vi "TDMS Numeric 2D Array to file.vi"(0 "Base path":path, 1 "Group Name":string="A", 2 "FileName":string, 3 "Interval":T1=enum."Daily", 5 "Channel Names":string[](array[string]), 9 "2D array":dbl[][](array[numeric]), 11 "error in (no error)":errorcluster, 12 "Channel Units":string[](array[string]), 13 "property Metadata":variant[](array[variant])) -> (4 "file out":refnum<k34>, 15 "error out":errorcluster)   [LabVIEW 2019]
doc: "This SubVI manages the TDMS write process for data formatted into string arrays. On first run or after a specified interval, it will create a new TDMS file with a unique file name utilizing the data and time when the file is created. During the first run, it will populate the metadata and unit fields of the TDMS header. After a specified interval of data streaming to the file, it will be closed and the file extension will be changed from .tdms to .done. This is feature is to assure file transfer functions don't grab files that are being actively written to (LabVIEW's TDMS Open vi does not allow custom/alternate/temp file extensions). File write buffers are automatically flushed every 60 seconds to assure minimal data loss in the event of a power failure or program interruption. \n\n\nThis vi differs from version 1 by adding inputs for writing to the units column in the metadata page. Will replace version 1 once other code is updated.\n\n2020 NREL"
uses:
  Enum_FileNewInterval.ctl
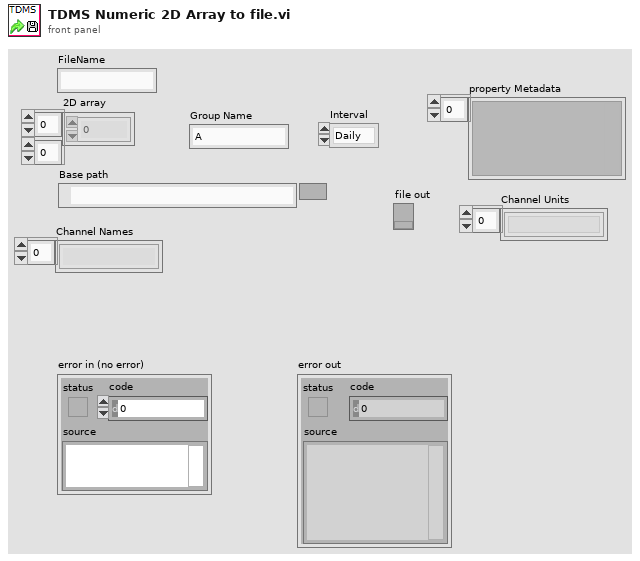
[diagram p1: front panel]
types:
  T1 = typedef "Enum_FileNewInterval.ctl" = enum16{"10 Min", "Hourly", "Daily", "Weekly", "Monthly"}
  T2 = enum16{"open", "open or create", "create or replace", "create", "open (read-only)"}
  T3 = typedef "LVDateTimeRec.ctl" = cluster{"fractional second":dbl, "second":i32, "minute":i32, "hour":i32, "day of month":i32, "month":i32, "year":i32, "day of week":i32, "day of year":i32, "DST":i32}
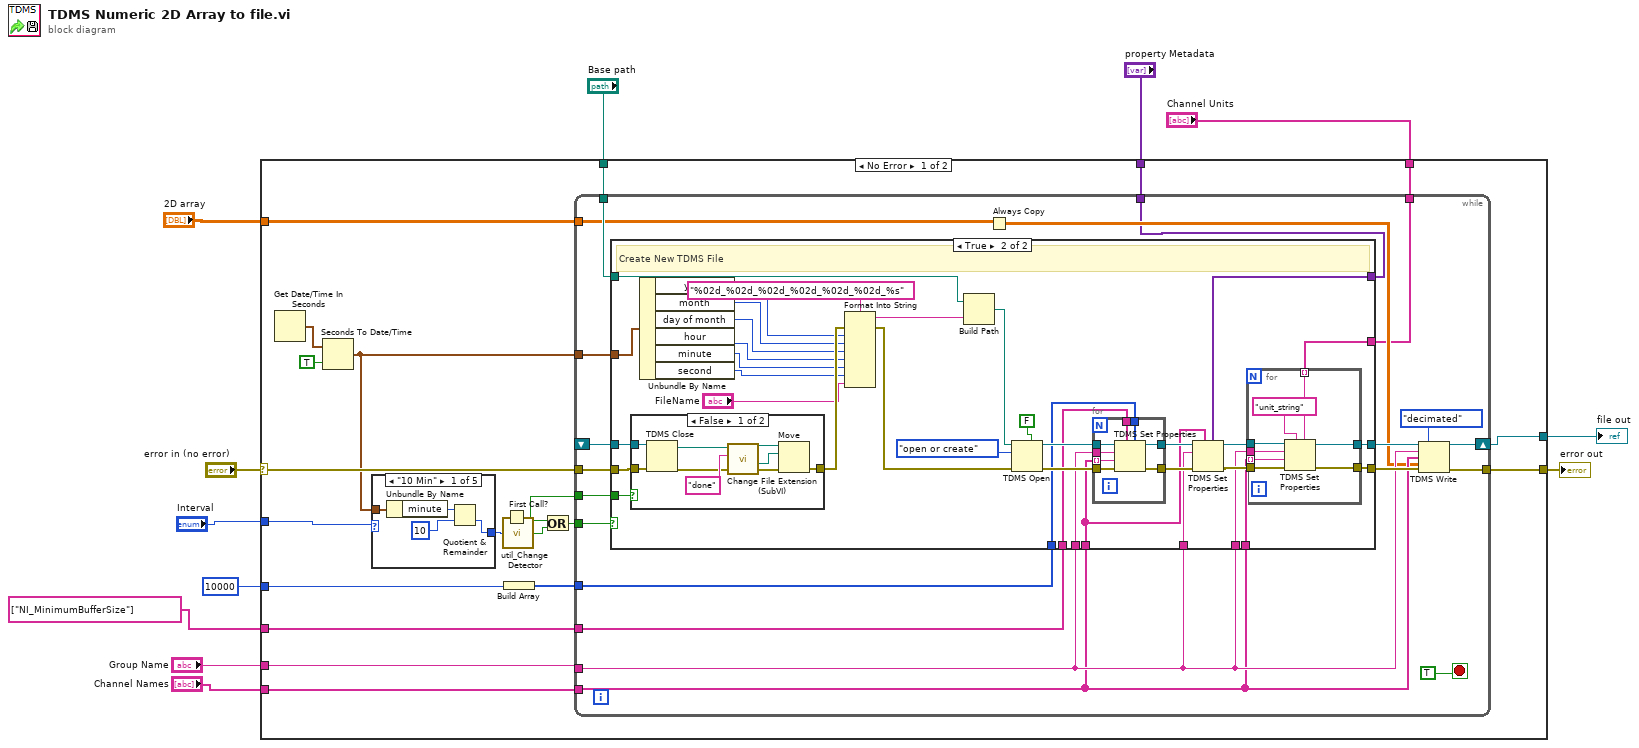
[diagram p0: block diagram]
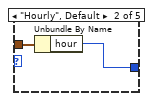
[diagram p2: hidden frame]
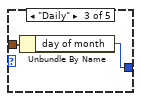
[diagram p3: hidden frame]
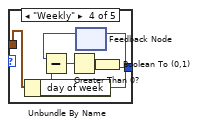
[diagram p4: hidden frame]
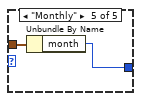
[diagram p5: hidden frame]
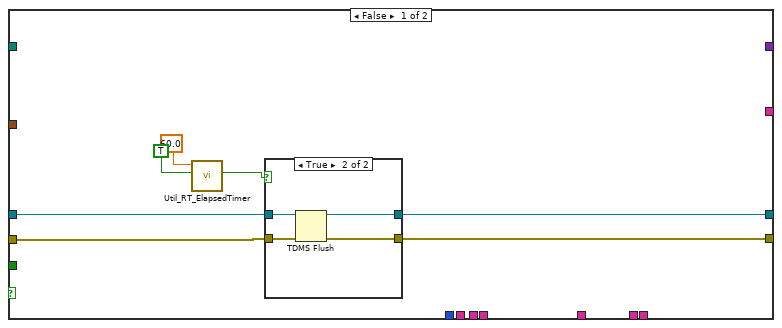
[diagram p6: hidden frame]
diagram:
  n1 = case shown="No Error" "error in (no error)" {
    selector: "error in (no error)" -> [w29 w143]
    tunnel: [w30 w143] -> w12
    tunnel: 10000 -> [w22 _]
    tunnel: "Interval" -> [w21 _]
    tunnel: string[] ["NI_MinimumBufferSize"] ("Channel Names") -> [w20 _]
    tunnel: "Channel Names" -> [w19 _]
    tunnel: "Group Name" -> [w18 _]
    tunnel: "Channel Units" -> [w17 _]
    tunnel: "property Metadata" -> [w16 _]
    tunnel: "Base path" -> [w15 _]
    tunnel: [w14 _] -> w2
    tunnel: "2D array" -> [w13 _]
    frame No Error {
      n2 = Get Date/Time In Seconds() -> (seconds since 1Jan1904=w26:timestamp)
      n3 = Seconds To Date/Time(time stamp (now)=w26, to UTC (F)=TRUE) -> (date time rec=w25:T3)
      n4 = case shown="\"10 Min\"" w21 {
        tunnel: w25 -> [w36 w38 w40 w46 w48]
        tunnel: [w33 w37 w39 w41 w47] -> w23
        frame "10 Min" {
          n5 = Unbundle By Name(w36) -> ("minute"=w35:i32)
          n6 = Quotient & Remainder(x=w35, y=10) -> (floor(x/y)=w33:i32)  [unwired: 1 out]
        }
        frame "Hourly", Default {
          n7 = Unbundle By Name(w38) -> ("hour"=w37:i32)
        }
        frame "Daily" {
          n8 = Unbundle By Name(w40) -> ("day of month"=w39:i32)
        }
        frame "Weekly" {
          n9 = Unbundle By Name(w46) -> ("day of week"=w44:i32)
          n10 = feedback-in #1(w44) -> ()
          n11 = feedback #1() -> (w45:i32)  [unwired: 1 in]
          n12 = Subtract(x=w45, y=w44) -> (x-y=w43:i32)
          n13 = Greater Than 0?(x=w43) -> (x > 0?=w42:bool)
          n14 = Boolean To (0,1)(Boolean=w42) -> (0, 1=w41:i16)
        }
        frame "Monthly" {
          n15 = Unbundle By Name(w48) -> ("month"=w47:i32)
        }
      }
      n16 = First Call?() -> (First Call?: T/F=w31:bool)
      n17 = call "util_Change Detector.vi"("value"=w23) -> ("changed?"=w24:bool)
      n18 = Build Array(w22) -> (w28:i32[])
      n19 = Or(x=w31, y=w24) -> (x .or. y?=w32:bool)
      n20 = while {
        tunnel: w32 -> [w68]
        shift-right: [w66] -> w14
        shift-left: _ -> [w67]
        tunnel: w31 -> [w65]
        tunnel: [w63] -> w30
        tunnel: w29 -> [w62]
        tunnel: w25 -> [w60]
        tunnel: w28 -> [w59]
        tunnel: w18 -> [w56]
        tunnel: w19 -> [w55]
        tunnel: w20 -> [w53]
        tunnel: w17 -> [w52]
        tunnel: w16 -> [w51]
        tunnel: w15 -> [w50]
        tunnel: w13 -> [w49]
        stop <- TRUE stop-if-true
        n21 = case shown="True" w68 {
          tunnel: w67 -> [w75 w112]
          tunnel: w65 -> [_ w113]
          tunnel: [w72 w90] -> w58
          tunnel: w62 -> [w73 w111]
          tunnel: w60 -> [_ w109]
          tunnel: [w74 w91] -> w57
          tunnel: w59 -> [_ w106]
          tunnel: w53 -> [_ w105]
          tunnel: w56 -> [_ w93]
          tunnel: w55 -> [_ w96]
          tunnel: w56 -> [_ w95]
          tunnel: w56 -> [_ w88]
          tunnel: w55 -> [_ w87]
          tunnel: w52 -> [_ w86]
          tunnel: w51 -> [_ w85]
          tunnel: w50 -> [_ w84]
          frame False {
            n22 = call "Util_RT_ElapsedTimer.vi"("Auto Reset"=TRUE, "Target Time (s)"=60.0) -> ("Target\nReached"=w69:bool)  [unwired: 8 in, 1 out]
            n23 = case shown="True" w69 {
              tunnel: w75 -> [w77 w81]
              tunnel: [w77 w80] -> w74
              tunnel: w73 -> [w76 w79]
              tunnel: [w76 w78] -> w72
              frame False {
              }
              frame True {
                n24 = TDMS Flush(4:w79, 7:w81) -> (0:w78:errorcluster, 3:w80:refnum<k34>)
              }
            }
          }
          frame True {
            # "Create New TDMS File"
            n25 = case shown="False" w113 {
              tunnel: w112 -> [w141 _]
              tunnel: [w137 w142] -> w117
              tunnel: w111 -> [w140 w142]
              frame False {
                n26 = TDMS Close(8:w140, 11:w141) -> (0:w136:errorcluster, 3:w135:path)
                n27 = call "Change File Extension (SubVI).vi"("New Extension"="done", "appended path"=w135) -> ("New file path"=w139:path, "Original Path"=w134:path)  [unwired: 7 in, 1 out]
                n28 = Move(source path=w134, error in=w136, 10:w139) -> (error out=w137:errorcluster)  [unwired: 2 in, 2 out]
              }
              frame True {
              }
            }
            n29 = Unbundle By Name(w109) -> ("year"=w103:i32, "month"=w102:i32, "day of month"=w101:i32, "hour"=w100:i32, "minute"=w99:i32, "second"=w82:i32)
            n30 = Format Into String(format string="%02d_%02d_%02d_%02d_%02d_%02d_%s", error in=w117, w103, w102, w101, w100, w99, w82, "FileName") -> (resulting string=w104:string, error out=w110:errorcluster)  [unwired: 1 in]
            n31 = Build Path(base path=w84, name or relative path=w104) -> (appended path=w115:path)
            n32 = TDMS Open(5:FALSE ("create index file? (T)"), 8:w110, 10:T2."open or create" ("operation (0:open)"), 11:w115) -> (0:w108:errorcluster, 3:w107:refnum<k34>)  [unwired: 3 in]
            n33 = for {
              tunnel: w107 -> [w133]
              tunnel: [w132] -> w98
              tunnel: w108 -> [w131]
              tunnel: [w130] -> w97
              tunnel: w105 -> [w129]
              tunnel: w106 -> [w128]
              tunnel: w93 -> [w127]
              tunnel: w96 -> [w126] mode=indexing
              n34 = TDMS Set Properties(5:w128, 7:w129, 8:w131, 9:w126, 10:w127, 11:w133) -> (0:w130:errorcluster, 3:w132:refnum<k34>)  [unwired: 2 out]
            }
            n35 = TDMS Set Properties(5:w85, 7:w96, 8:w97, 10:w95, 11:w98) -> (0:w89:errorcluster, 3:w92:refnum<k34>)  [unwired: 1 in, 2 out]
            n36 = for {
              tunnel: w88 -> [w123]
              tunnel: w92 -> [w125]
              tunnel: [w124] -> w91
              tunnel: [w122] -> w90
              tunnel: w89 -> [w121]
              tunnel: w87 -> [w120] mode=indexing
              tunnel: w86 -> [w118] mode=indexing
              n37 = TDMS Set Properties(5:w118, 7:"unit_string", 8:w121, 9:w120, 10:w123, 11:w125) -> (0:w122:errorcluster, 3:w124:refnum<k34>)  [unwired: 2 out]
            }
          }
        }
        n38 = Always Copy(1:w49) -> (0:w54:dbl[][])
        n39 = TDMS Write(0:w57, 1:enum16{"decimated", "interleaved"}."decimated" ("data layout (0:decimated)"), 5:w56, 7:w55, 9:w54, 11:w58) -> (4:w66:refnum<k34>, 15:w63:errorcluster)  [unwired: 2 out]
      }
    }
    frame Error {
    }
  }
  "error out" <- w12
  "file out" <- w2
